vi "Set_Coh_Control_Status.vi"(0 ".NET Reference in":refnum<k24>, 1 "status":i32(ring) items=["Coh_OFF", "Coh_ON"], 3 "error in (no error)":errorcluster) -> (7 "Reference out":refnum<k24>, 10 "error out":errorcluster)   [LabVIEW 2017]
uses:
  C:/Users/Ssantec_Test/Documents/Instrument_DLL_Sample_Labview_20220902_Ver1.2.2/DLL/x86/InstrumentDLL.dll
  DLL/x86/InstrumentDLL.dll
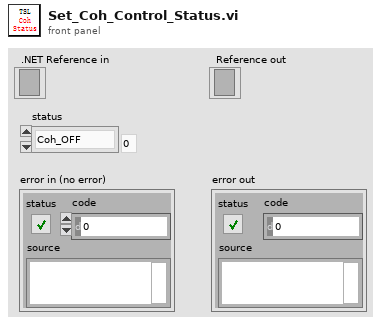
[diagram p1: front panel]
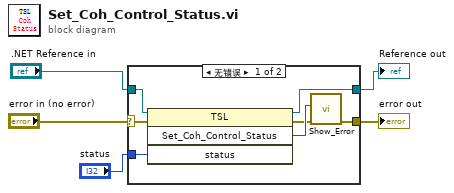
[diagram p0: block diagram]
diagram:
  n1 = case shown="无错误" "error in (no error)" {
    selector: "error in (no error)" -> [w6 w14]
    tunnel: "status" -> [w12 _]
    tunnel: ".NET Reference in" -> [w11 w13]
    tunnel: [w10 w13] -> w4
    tunnel: [w7 w14] -> w3
    frame No Error {
      n2 = invoke on="调用节点" class="TSL" method="Set_Coh_Control_Status"(reference=w11, error in=w6, "status"=w12) -> (reference out=w10:refnum<k24>, error out=w8:errorcluster, "Set_Coh_Control_Status"=w9:i32)  [unwired: 1 in, 1 out]
      n3 = call "Show_Error.vi"("error in (no error)"=w8, "Error"=w9) -> ("error out"=w7:errorcluster)  [unwired: 9 in]
    }
    frame Error {
    }
  }
  "Reference out" <- w4
  "error out" <- w3
